vi "jsonToTest.vi"(8 "error in (no error)":errorcluster, 11 "JSON string":string) -> (0 "error out":errorcluster, 3 "Tests":refnum<class "TestInterface.lvclass">[](array[class]))   [LabVIEW 2013, in "DataCreation.lvlib"]
doc: "Wandelt einen JSON-String in ein Test-Objekte-Array um"
uses:
  classes/Tests/TestInterface/TestInterface.lvclass
  classes/Tests/Stoeraussendung/Stoeraussendung.lvclass
  classes/Tests/Burst/Burst.lvclass
  classes/Tests/ESD/ESD.lvclass
  classes/Tests/Surge/Surge.lvclass
  classes/Tests/Spannungseinbruch/Spannungseinbruch.lvclass
  classes/Tests/HF-Felder/HF-Felder.lvclass
  lib/DataCreation.lvlib
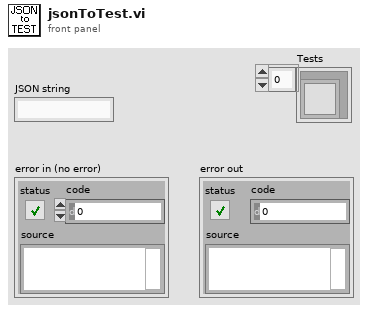
[diagram p1: front panel]
types:
  T1 = cluster{"class name":string, "Command regex":string[], "Commandlist":string, "name":string, "response":bool[], "timings":i32[], "wait":u32[], "parameter table":string[][], "parameters":string[]}[]
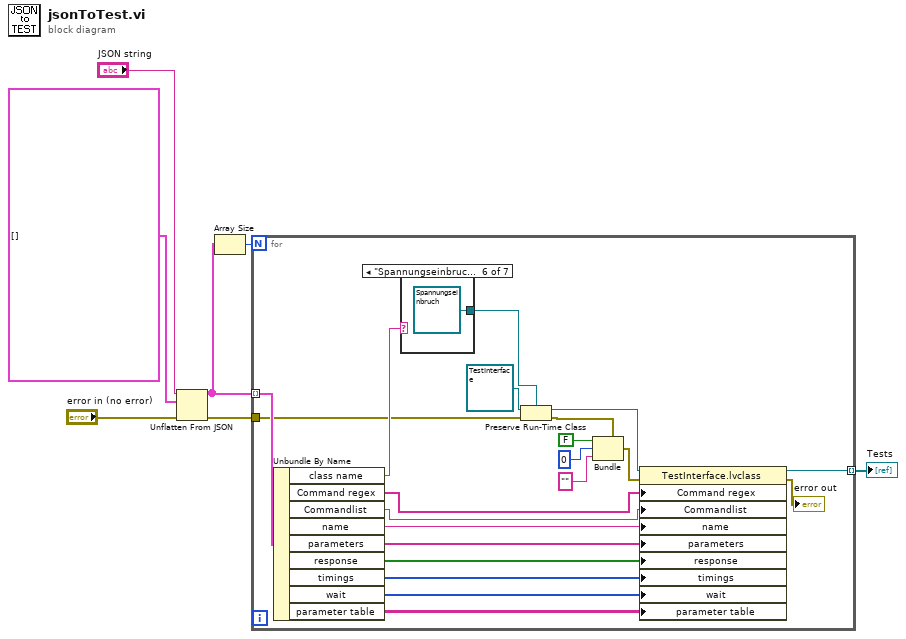
[diagram p0: block diagram]
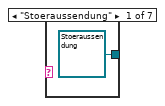
[diagram p2: hidden frame]
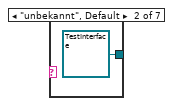
[diagram p3: hidden frame]
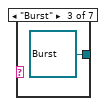
[diagram p4: hidden frame]
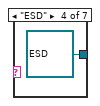
[diagram p5: hidden frame]
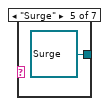
[diagram p6: hidden frame]
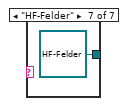
[diagram p7: hidden frame]
diagram:
  n1 = Unflatten From JSON(JSON string="JSON string", type and defaults=T1 [] ("appended array"), error in (no error)="error in (no error)") -> (value=w3:T1, error out=w4:errorcluster)  [unwired: 4 in]
  n2 = Array Size(array=w3) -> (size(s)=w2:i32)
  n3 = for {
    N: w2 -> [_]
    tunnel: w3 -> [w12] mode=indexing
    tunnel: w4 -> [w11]
    tunnel: [w10] -> w1 mode=indexing
    n4 = Unbundle By Name(w12) -> ("class name"=w25:string, "Command regex"=w19:string[], "Commandlist"=w18:string, "name"=w17:string, "parameters"=w9:string[], "response"=w16:bool[], "timings"=w15:i32[], "wait"=w14:u32[], "parameter table"=w8:string[][])
    n5 = case shown="\"Spannungseinbruch\"" w25 {
      tunnel: [refnum<class "Stoeraussendung.lvclass"> refnum ("Störaussendung.lvclass") refnum<class "TestInterface.lvclass"> refnum ("Burst.lvclass") refnum<class "Burst.lvclass"> refnum ("Burst.lvclass") refnum<class "ESD.lvclass"> refnum ("ESD.lvclass") refnum<class "Surge.lvclass"> refnum ("Surge.lvclass") refnum<class "Spannungseinbruch.lvclass"> refnum ("Spannungseinbruch.lvclass") refnum<class "HF-Felder.lvclass"> refnum ("HF-Felder.lvclass")] -> w28
      frame "Stoeraussendung" {
      }
      frame "unbekannt", Default {
      }
      frame "Burst" {
      }
      frame "ESD" {
      }
      frame "Surge" {
      }
      frame "Spannungseinbruch" {
      }
      frame "HF-Felder" {
      }
    }
    n6 = Preserve Run-Time Class(object in=refnum<class "TestInterface.lvclass"> refnum ("TestInterface.lvclass"), error in=w11, 2:w28) -> (object out=w26:refnum<class "TestInterface.lvclass">, error out=w21:errorcluster)
    n7 = Bundle(cluster=w21, "status"=FALSE, "code"=0, "source"="") -> (w20:errorcluster)
    n8 = property class="TestInterface.lvclass"(reference=w26, error in=w20, "Command regex"=w19, "Commandlist"=w18, "name"=w17, "parameters"=w9, "response"=w16, "timings"=w15, "wait"=w14, "parameter table"=w8) -> (reference out=w10:refnum<class "TestInterface.lvclass">, error out=→"error out":errorcluster)
  }
  "Tests" <- w1
